vi "live_scanner.vi"(0 "live_pixel_dwell_ms":dbl=0.1 caption="Dwell time:", 1 "pos-start_x":refnum<vi>, 2 "pos-start_y":refnum<vi>, 3 "enable":refnum<vi>, 5 "live_frame_size_x_px":i32=50 caption="image_size_x", 7 "image_size_x_um":dbl=6.0, 9 "pos_start":enum32{"bottom-left", "center"}(ring), 11 "live_scan_direction":enum32{"0", "1"}(radio)=enum."1" caption="Scan direction:", 12 "IntensityGraph in":refnum<vi>) -> (6 "image_out":dbl[][](array[numeric]))   [LabVIEW 2014]
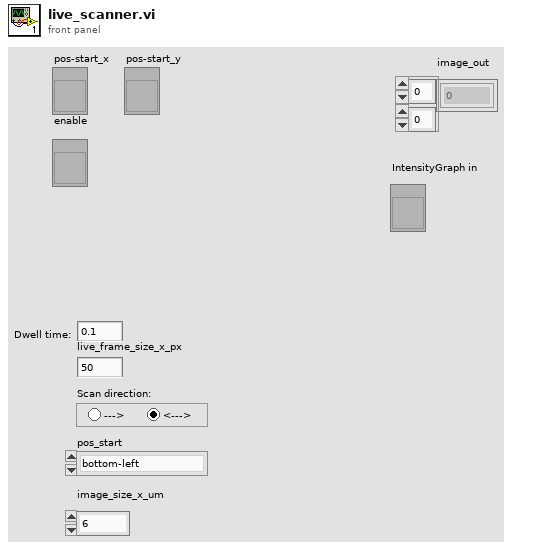
[diagram p1: front panel]
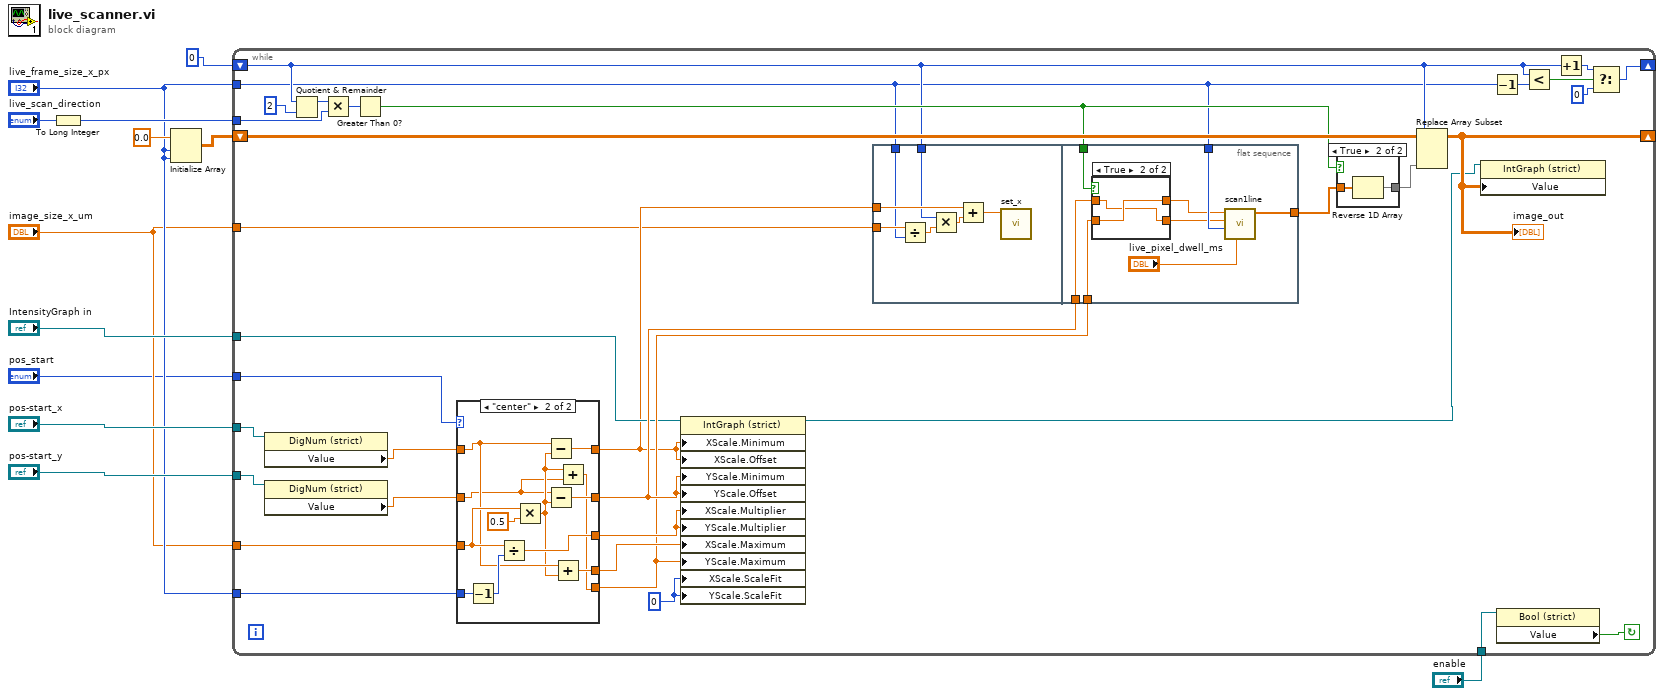
[diagram p0: block diagram]
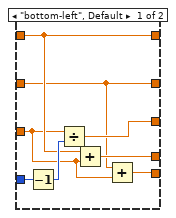
[diagram p4: hidden frame]
diagram:
  n1 = To Long Integer(number="live_scan_direction") -> (32bit integer=w4:i32)
  n2 = Initialize Array(0.0 ("element"), "live_frame_size_x_px", "live_frame_size_x_px") -> (w10:dbl[][])
  n3 = while {
    shift-right: [w45] -> _
    shift-left: w10 -> [w46]
    shift-right: [w44] -> _
    shift-left: 0 -> [w20]
    tunnel: "live_frame_size_x_px" -> [w19]
    tunnel: "pos-start_x" -> [w27]
    tunnel: "pos-start_y" -> [w26]
    tunnel: "image_size_x_um" -> [w15]
    tunnel: "enable" -> [w25]
    tunnel: "IntensityGraph in" -> [w23]
    tunnel: w4 -> [w22]
    tunnel: "live_frame_size_x_px" -> [w17]
    tunnel: "image_size_x_um" -> [w16]
    tunnel: "pos_start" -> [w14]
    stop <- w24 continue-if-true
    w13 = u8 0 ("X Scale.Scale Fit")
    n4 = property on="Property Node" class="DigNum (strict)"(reference=w27) -> ("Value"=w39:dbl)  [unwired: 1 in, 2 out]
    n5 = property on="Property Node" class="DigNum (strict)"(reference=w26) -> ("Value"=w38:dbl)  [unwired: 1 in, 2 out]
    n6 = Quotient & Remainder(x=w20, y=2) -> (x-y*floor(x/y)=w34:i32)  [unwired: 1 out]
    n7 = Multiply(x=w34, y=w22) -> (x*y=w33:i32)
    n8 = Greater Than 0?(x=w33) -> (x > 0?=w30:bool)
    n9 = case shown="\"center\"" w14 {
      tunnel: w39 -> [w73 w82]
      tunnel: w38 -> [w70 w79]
      tunnel: w15 -> [w71 w86]
      tunnel: [w73 w83] -> w21
      tunnel: [w70 w84] -> w29
      tunnel: [w75 w87] -> w37
      tunnel: [w74 w81] -> w36
      tunnel: [w72 w78] -> w28
      tunnel: w17 -> [w69 w77]
      frame "bottom-left", Default {
        n10 = Decrement(x=w69) -> (x-1=w76:i32)
        n11 = Divide(x=w71, y=w76) -> (x/y=w75:dbl)
        n12 = Add(x=w73, y=w71) -> (x+y=w74:dbl)
        n13 = Add(x=w70, y=w71) -> (x+y=w72:dbl)
      }
      frame "center" {
        n14 = Decrement(x=w77) -> (x-1=w88:i32)
        n15 = Divide(x=w86, y=w88) -> (x/y=w87:dbl)
        n16 = Multiply(x=w86, y=0.5) -> (x*y=w80:dbl)
        n17 = Subtract(x=w82, y=w80) -> (x-y=w83:dbl)
        n18 = Subtract(x=w79, y=w80) -> (x-y=w84:dbl)
        n19 = Add(x=w82, y=w80) -> (x+y=w81:dbl)
        n20 = Add(x=w80, y=w79) -> (x+y=w78:dbl)
      }
    }
    n21 = property on="Property Node" class="IntGraph (strict)"(reference=w23, "XScale.Minimum"=w21, "XScale.Offset"=w21, "YScale.Minimum"=w29, "YScale.Offset"=w29, "XScale.Multiplier"=w37, "YScale.Multiplier"=w37, "XScale.Maximum"=w36, "YScale.Maximum"=w28, "XScale.ScaleFit"=w13, "YScale.ScaleFit"=w13) -> (reference out=w18:refnum<vi>)  [unwired: 1 in, 1 out]
    n22 = flat-sequence {
      tunnel: w21 -> [w53]
      tunnel: w20 -> [w51]
      tunnel: w16 -> [w49]
      tunnel: w19 -> [w48]
      tunnel: [w60] -> w32
      tunnel: w19 -> [w59]
      tunnel: w30 -> [w56]
      tunnel: w29 -> [w55]
      tunnel: w28 -> [w54]
      frame #0 {
        n23 = Divide(x=w49, y=w48) -> (x/y=w50:dbl)
        n24 = Multiply(x=w51, y=w50) -> (x*y=w52:dbl)
        n25 = Add(x=w53, y=w52) -> (x+y=w47:dbl)
        n26 = call "set_x.vi"("x_value_um"=w47) -> ()  [unwired: 10 in, 1 out]
      }
      frame #1 {
        n27 = case shown="True" w56 {
          tunnel: [w62 w65] -> w58
          tunnel: [w63 w64] -> w57
          tunnel: w54 -> [w63 w65]
          tunnel: w55 -> [w62 w64]
          frame False {
          }
          frame True {
          }
        }
        n28 = call "scan1line.vi"("dwell_time_ms"="live_pixel_dwell_ms", "q_pixels"=w59, "y_end"=w57, "y_start"=w58) -> ("histogram plot"=w60:dbl[])  [unwired: 6 in, 1 out]
      }
    }
    n29 = case shown="True" w30 {
      tunnel: w32 -> [w66 w68]
      tunnel: [w66 w67] -> w31
      frame False {
      }
      frame True {
        n30 = Reverse 1D Array(array=w68) -> (reversed array=w67:dbl[])
      }
    }
    n31 = Replace Array Subset(array=w46, new element=w31, index (row)=w20) -> (w45:dbl[][])  [unwired: 1 in]
    "image_out" <- w45
    n32 = property on="Property Node" class="IntGraph (strict)"(reference=w18, "Value"=w45) -> ()  [unwired: 1 in, 2 out]
    n33 = Decrement(x=w19) -> (x-1=w40:i32)
    n34 = property class="Bool (strict)"(reference=w25) -> ("Value"=w24:bool)  [unwired: 1 in, 2 out]
    n35 = Less?(x=w20, y=w40) -> (x < y?=w41:bool)
    n36 = Increment(x=w20) -> (x+1=w43:i32)
    n37 = Select(t=w43, s=w41, f=0) -> (s? t:f=w44:i32)
  }
